vi "SendTo_Queue.vi"(8 "Max Queue Size":i32=-1, 9 "Timeout (ms)":i32=-1, 10 "Message":variant, 11 "Queue Name":string) -> (3 "Node Out":refnum<class "bt_Node.lvclass">)   [LabVIEW 2021, in "BT.lvlib"]
uses:
  BT.lvlib
  Support/Nodes/Leaves/Synch/With Values/Send/bt_Send_Synch_WithValues.lvclass/bt_Send_Synch_WithValues.ctl
  Support/Nodes/Leaves/Synch/Queue/Send/bt_Send_Queue.lvclass/bt_Send_Queue.ctl
  Support/Nodes/Leaves/Synch/With Values/Send/Properties/Write Values.vi
  Support/Nodes/Leaves/Synch/Queue/Send/Properties/Write Name.vi
  Support/Nodes/Leaves/Synch/Queue/Send/Properties/Write max queue size.vi
  Support/Nodes/Leaves/Synch/Queue/Send/Properties/Write timeout.vi
  Support/Nodes/Leaves/Synch/Queue/Send/bt_Send_Queue.lvclass
  C:/Users/Tim/Documents/GitHub/LV_Behaviour_Tree/Source/Support/Nodes/Leaves/Synch/With Values/Send/bt_Send_Synch_WithValues.lvclass
  C:/Users/Tim/Documents/GitHub/LV_Behaviour_Tree/Source/Support/Nodes/Leaves/Synch/Parent/Send/bt_Send_Synch.lvclass
  C:/Users/Tim/Documents/GitHub/LV_Behaviour_Tree/Source/Support/Nodes/Leaves/Leaf/bt_Leaf.lvclass
  C:/Users/Tim/Documents/GitHub/LV_Behaviour_Tree/Source/Support/Nodes/abs_Node/bt_Node.lvclass
  C:/Users/Tim/Documents/GitHub/LV_Behaviour_Tree/Source/Support/Nodes/Leaves/Synch/Queue/Send/bt_Send_Queue.lvclass
  Support/Nodes/abs_Node/bt_Node.lvclass
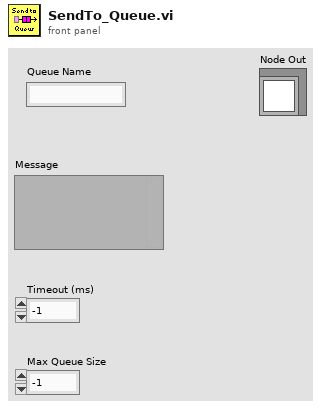
[diagram p1: front panel]
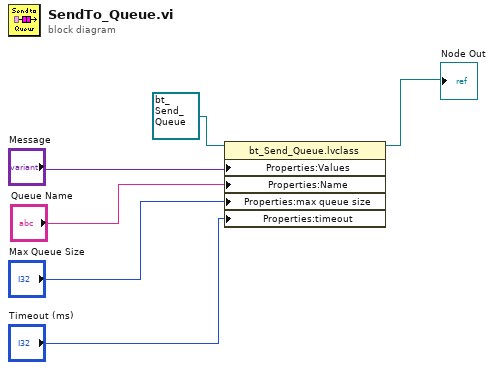
[diagram p0: block diagram]
diagram:
  n1 = property class="bt_Send_Queue.lvclass"(reference=refnum<class "bt_Send_Queue.lvclass"> refnum ("BT.lvlib:bt_Send_Queue.lvclass"), "Properties:Values"="Message", "Properties:Name"="Queue Name", "Properties:max queue size"="Max Queue Size", "Properties:timeout"="Timeout (ms)") -> (reference out=→"Node Out":refnum<class "bt_Send_Queue.lvclass">)  [unwired: 1 in, 1 out]
